vi "NI_DAQ_Create.vi"(0 "reference in":refnum<class "NI_DAQ.lvclass">, 5 "error in (no error)":errorcluster) -> (14 "reference out":refnum<class "NI_DAQ.lvclass">, 19 "error out":errorcluster)   [LabVIEW 2020, in "DAQ.lvlib" / "NI_DAQ.lvclass"]
doc: "Constructor."
uses:
  NI_DAQ.lvclass
  C:/Program Files (x86)/National Instruments/LabVIEW 2020/vi.lib/addons/_AddQ/G#Object/G#Object.lvclass
  D:/BingoGithub/DAQ_V000.01/DAQ_Base_class/DAQ_Base.lvclass
  <vilib>/addons/_AddQ/G#Object/G#Object.lvclass
  DAQ_Base_class/DAQ_Base.lvclass
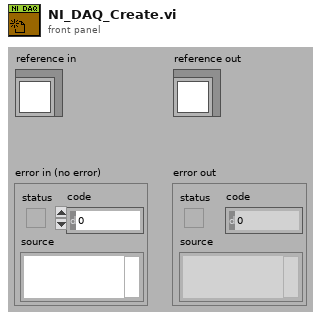
[diagram p1: front panel]
types:
  T1 = typedef "DAQ.lvlib/NI_DAQ.lvclass/ObjectAttributesRef.ctl" = refnum<data-value>
  T2 = typedef "DAQ.lvlib/NI_DAQ.lvclass/ObjectAttributes.ctl" = cluster{"MyAttribute":dbl, "DAQ_AI_task_out":refnum<k21>, "counter_task_out":refnum<k21>[]}
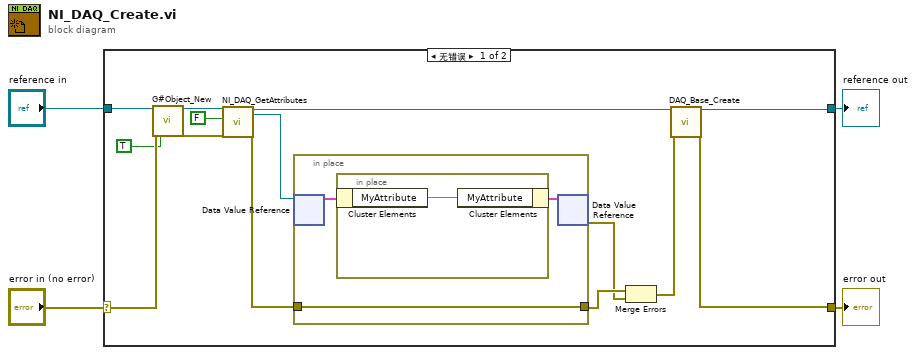
[diagram p0: block diagram]
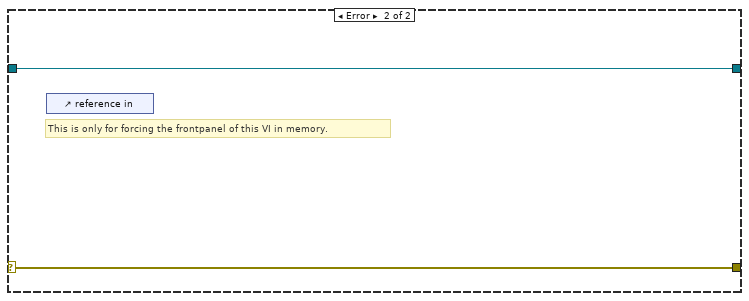
[diagram p2: hidden frame]
diagram:
  n1 = case shown="无错误" "error in (no error)" {
    selector: "error in (no error)" -> [w17 w24]
    tunnel: [w5 w24] -> w3
    tunnel: [w7 w23] -> w1
    tunnel: "reference in" -> [w18 w23]
    frame No Error {
      n2 = call <vilib>:"G#Object_New.vi"("reference in"=w18, "error in (no error)"=w17, "user counter (T)?"=TRUE ("User Counter")) -> ("reference out"=w10:refnum<class "NI_DAQ.lvclass">, "error out"=w9:errorcluster)  [unwired: 14 in, 1 out]
      n3 = call "NI_DAQ_GetAttributes.vi"("reference in"=w10, "return data? (T)"=FALSE ("return data"), "error in (no error)"=w9) -> ("reference out"=w8:refnum<class "NI_DAQ.lvclass">, "attributes ref"=w12:T1, "error out"=w13:errorcluster)  [unwired: 13 in, 1 out]
      n4 = in-place {
        in-place-border: w13 -> [w19]
        in-place-border: [w19] -> w15
        n5 = in-place-dvr #1(w12) -> (w20:T2)  [unwired: 1 out]
        n6 = in-place {
          n7 = in-place-cluster #2(w20) -> ("MyAttribute"=w22:dbl)
          n8 = in-place-cluster #2("MyAttribute"=w22) -> (w21:T2)
        }
        n9 = in-place-dvr #1(w21) -> (w14:errorcluster)  [unwired: 1 out]
      }
      n10 = Merge Errors(w15, w14) -> (w6:errorcluster)
      n11 = call "DAQ_Base_Create.vi"("reference in"=w8, "error in (no error)"=w6) -> ("reference out"=w7:refnum<class "NI_DAQ.lvclass">, "error out"=w5:errorcluster)  [unwired: 16 in]
    }
    frame Error {
      # "This is only for forcing the frontpanel of this VI in memory."
      n12 = control-ref of="reference in"() -> ()  [unwired: 1 out]
    }
  }
  "error out" <- w3
  "reference out" <- w1
